vi "RTM Add Waveforms.vi"(8 "error in (no error)":errorcluster, 11 "Node Ptr":u64 format="%.0x") -> (0 "error out":errorcluster)   [LabVIEW 2015]
uses:
  NationalInstruments.VeriStand.SystemStorage
  <vilib>/NI VeriStand/UI Controls/System Definition Tree/NI_VS UI System Tree.lvlib
  NationalInstruments.VeriStand.SystemStorageUI
  <vilib>/NI VeriStand/Custom Device API/Custom Device API.lvlib
  Waveform-Processing-Custom-Device System Explorer.lvlib
panel:
  in  "OK Button":bool
  in  "TreeBrowserWF":refnum<k24>(container)
  in  "Tag":string
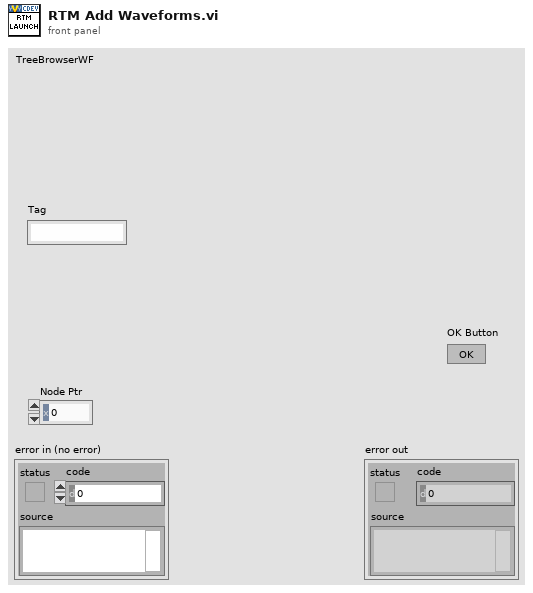
[diagram p1: front panel]
types:
  T1 = typedef "Custom Device API.lvlib/Custom Device Item Ref.ctl" = u64
  T2 = typedef "Custom Device API.lvlib/Custom Device Pointer.ctl" = refnum<k24>
  T3 = typedef "NI_VS UI System Tree.lvlib/Callback Type.ctl" = cluster{"Net Callbacks":refnum<k27>[], "Event":T4}
  T4 = typedef "NI_VS UI System Tree.lvlib/Net Event Data Ref.ctl" = refnum<user-event>
  T5 = typedef "NI_VS UI System Tree.lvlib/System Definition Tree Ref.ctl" = refnum<k24>
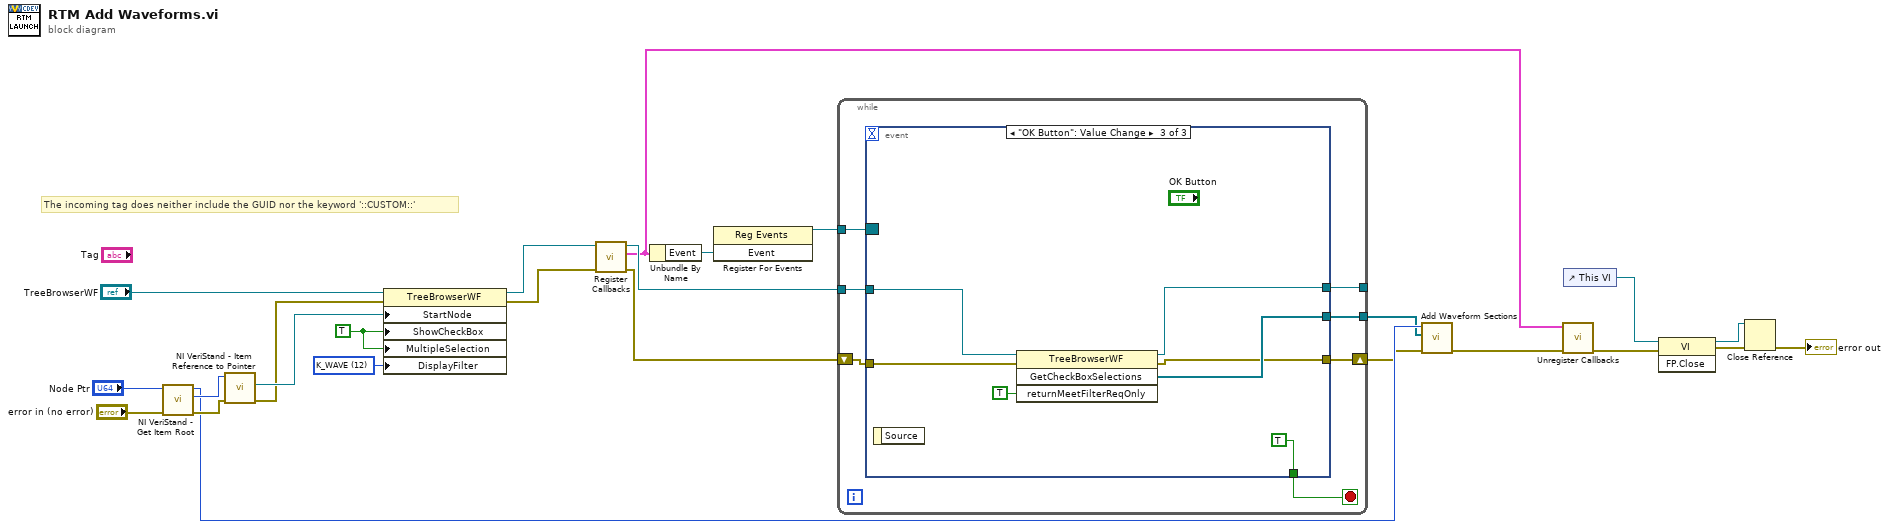
[diagram p0: block diagram]
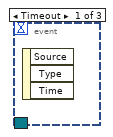
[diagram p2: hidden frame]
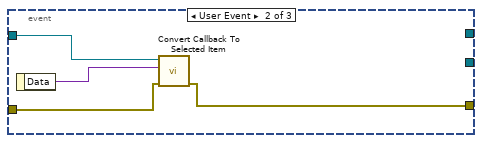
[diagram p3: hidden frame]
diagram:
  w10 = u8 12 items=["K_CHAN_R", "K_CHAN_W", "K_CHAN_RW", "K_CHAN_VOLT", "K_CHAN_FAULT", "K_ALL", "K_CUSTOM", "K_CHAN_R_VIS", "K_CHAN_W_VIS", "K_CHAN_RW_VIS", "K_CHAN_VOLT_VIS", "K_CHAN_FAULT_VIS", "K_WAVE", "K_WAVE_VIS", "K_WAVE_DBL", "K_WAVE_CDB", "K_WAVE_DBL_VIS", "K_WAVE_CDB_VIS"] ("DisplayFilter")
  w11 = TRUE ("ShowCheckBox")
  # "The incoming tag does neither include the GUID nor the keyword '::CUSTOM::'"
  n1 = call <vilib>:"NI VeriStand - Get Item Root.vi"("error in (no error)"="error in (no error)", "Item Ref in"="Node Ptr") -> ("error out"=w13:errorcluster, "Root Ref out"=w18:T1, "Item Ref out"=w9:T1)  [unwired: 6 in, 1 out]
  n2 = call <vilib>:"NI VeriStand - Item Reference to Pointer.vi"("error in (no error)"=w13, "Item Ref in"=w18) -> ("error out"=w12:errorcluster, "Node Pointer"=w17:T2)  [unwired: 6 in, 2 out]
  n3 = property class="TreeBrowserWF"(reference="TreeBrowserWF", error in=w12, "StartNode"=w17, "ShowCheckBox"=w11, "MultipleSelection"=w11, "DisplayFilter"=w10) -> (reference out=w15:refnum<k24>, error out=w16:errorcluster)
  n4 = call <vilib>:"Register Callbacks.vi"("error in (no error)"=w16, "System Definition Tree"=w15) -> ("error out"=w24:errorcluster, "Callbacks"=w22:T3, "System Definition Tree dup"=w23:T5)  [unwired: 7 in]
  n5 = Unbundle By Name(w22) -> ("Event"=w21:T4)
  n6 = register-events(w21) -> (reference out=w25:refnum<event-registration>)  [unwired: 2 in, 1 out]
  n7 = while {
    tunnel: w25 -> [w32]
    tunnel: w23 -> [w30]
    shift-right: [w29] -> w7
    shift-left: w24 -> [w31]
    tunnel: [w27] -> _
    tunnel: [w26] -> w8
    stop <- w28 stop-if-true
    n8 = event shown="[2] \"OK Button\": Value Change" {
      selector: w32 -> [_ _ _]
      dyn-events: _ -> [_ _ _]
      timeout: _ -> [_ _ _]
      tunnel: w31 -> [_ w35 w41]
      tunnel: w30 -> [_ w34 w42]
      tunnel: [_ w33 w38] -> w29
      tunnel: [_ _ TRUE] -> w28
      tunnel: [_ _ w40] -> w27
      tunnel: [_ _ w39] -> w26
      event Timeout {
        n9 = event-data() -> ()  [unwired: 1 in, 3 out]
      }
      event User Event {
        n10 = event-data() -> ("Data"=w36:variant)  [unwired: 1 in]
        n11 = call <vilib>:"Convert Callback To Selected Item.vi"("error in"=w35, "Data"=w36, "SystemDefinitionBrowser Ref"=w34) -> ("error out"=w33:errorcluster)  [unwired: 7 in, 1 out]
      }
      event "OK Button": Value Change {
        n12 = event-data() -> ()  [unwired: 1 in, 1 out]
        n13 = invoke class="TreeBrowserWF" method="GetCheckBoxSelections"(reference=w42, error in=w41, "returnMeetFilterReqOnly"=TRUE) -> (reference out=w40:T5, error out=w38:errorcluster, "GetCheckBoxSelections"=w39:refnum<k24>[])  [unwired: 1 in, 1 out]
      }
    }
  }
  n14 = call "Add Waveform Sections.vi"("error in"=w7, "Wfm Pointers"=w8, "CustomDevice Ref"=w9) -> ("error out"=w6:errorcluster)  [unwired: 7 in, 1 out]
  n15 = call <vilib>:"Unregister Callbacks.vi"("error in (no error)"=w6, "Callbacks"=w22) -> ("error out"=w2:errorcluster)  [unwired: 9 in]
  n16 = control-ref of="This VI"() -> (w5:refnum<vi>)
  n17 = invoke class="VI" method="FP.Close"(reference=w5, error in=w2) -> (reference out=w3:refnum<vi>, error out=w4:errorcluster)  [unwired: 1 in, 1 out]
  n18 = Close Reference(reference=w3, error in (no error)=w4) -> (error out=→"error out":errorcluster)
